vi "Fix Range on Representation Change.vi"(8 "error in (no error)":errorcluster, 11 "Numeric Data Type in":refnum<class "Numeric Data Type.lvclass">) -> (0 "error out":errorcluster, 3 "Numeric Data Type out":refnum<class "Numeric Data Type.lvclass">)   [LabVIEW 2018, in "Numeric Data Type.lvclass"]
uses:
  Numeric Data Type.lvclass
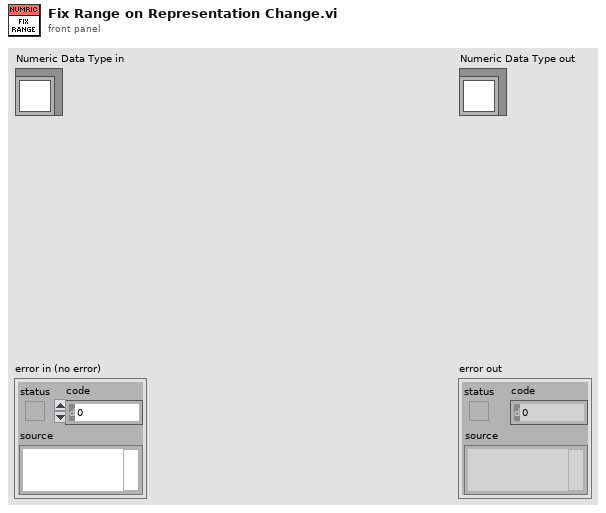
[diagram p1: front panel]
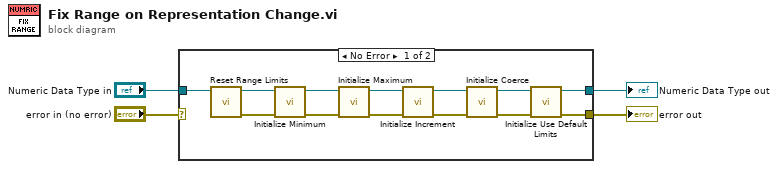
[diagram p0: block diagram]
diagram:
  n1 = case shown="No Error" "error in (no error)" {
    selector: "error in (no error)" -> [_ w19]
    tunnel: [w8 w19] -> w3
    tunnel: [w10 w18] -> w1
    tunnel: "Numeric Data Type in" -> [w7 w18]
    frame No Error {
      n2 = call "Reset Range Limits.vi"("Numeric Data Type in"=w7) -> ("error out"=w5:errorcluster, "Numeric Data Type out"=w6:refnum<class "Numeric Data Type.lvclass">)  [unwired: 9 in]
      n3 = call "Initialize Minimum.vi"("error in (no error)"=w5, "Numeric Data Type in"=w6) -> ("error out"=w15:errorcluster, "Numeric Data Type (dup)"=w17:refnum<class "Numeric Data Type.lvclass">)  [unwired: 8 in]
      n4 = call "Initialize Maximum.vi"("error in (no error)"=w15, "Numeric Data Type in"=w17) -> ("error out"=w14:errorcluster, "Numeric Data Type (dup)"=w16:refnum<class "Numeric Data Type.lvclass">)  [unwired: 8 in]
      n5 = call "Initialize Increment.vi"("error in (no error)"=w14, "Numeric Data Type in"=w16) -> ("error out"=w12:errorcluster, "Numeric Data Type (dup)"=w13:refnum<class "Numeric Data Type.lvclass">)  [unwired: 8 in]
      n6 = call "Initialize Coerce.vi"("error in (no error)"=w12, "Numeric Data Type in"=w13) -> ("error out"=w9:errorcluster, "Numeric Data Type (dup)"=w11:refnum<class "Numeric Data Type.lvclass">)  [unwired: 8 in]
      n7 = call "Initialize Use Default Limits.vi"("error in (no error)"=w9, "Numeric Data Type in"=w11) -> ("error out"=w8:errorcluster, "Numeric Data Type (dup)"=w10:refnum<class "Numeric Data Type.lvclass">)  [unwired: 8 in]
    }
    frame Error {
    }
  }
  "error out" <- w3
  "Numeric Data Type out" <- w1
